vi "Immediate Shot Distance.vi"() -> (1 "Pointed At Goal?":bool, 2 "Aimpoint X":dbl, 3 "Aimpoint Distance":dbl)   [LabVIEW 2013]
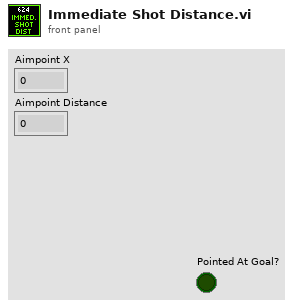
[diagram p1: front panel]
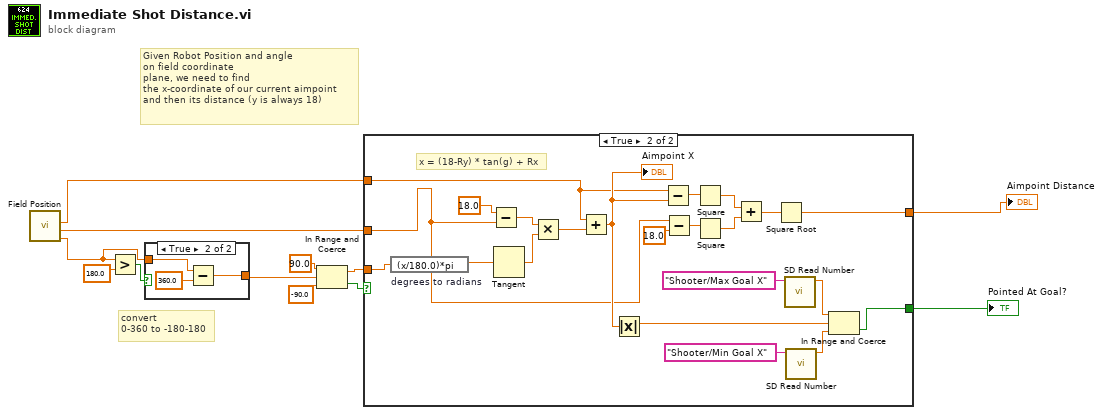
[diagram p0: block diagram]
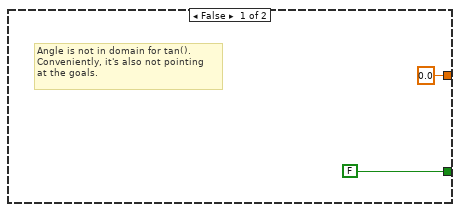
[diagram p2: hidden frame]
diagram:
  # "convert \n0-360 to -180-180"
  # "Given Robot Position and angle\non field coordinate\nplane, we need to find \nthe x-coordinate of our current aimpoint\nand then its distance (y is always 18)"
  n1 = call "Field Position.vi"() -> ("Field Angle"=w3:dbl, "Field Y"=w1:dbl, "Field X"=w2:dbl)  [unwired: 8 in, 1 out]
  n2 = Greater?(x=w3, y=180.0) -> (0:w11:bool)
  n3 = case shown="True" w11 {
    tunnel: w3 -> [w13 w16]
    tunnel: [w13 w14] -> w10
    frame False {
    }
    frame True {
      n4 = Subtract(x=w16, y=360.0) -> (x-y=w14:dbl)
    }
  }
  n5 = In Range and Coerce(upper limit=90.0, x=w10, lower limit=-90.0) -> (coerced(x)=w5:dbl, In Range?=w7:bool)
  n6 = case shown="True" w7 {
    tunnel: [FALSE w21] -> w6
    tunnel: w5 -> [_ w38]
    tunnel: [0.0 w27] -> w4
    tunnel: w2 -> [_ w20]
    tunnel: w1 -> [_ w19]
    frame False {
      # "Angle is not in domain for tan().\nConveniently, it's also not pointing\nat the goals."
    }
    frame True {
      # "x = (18-Ry) * tan(g) + Rx"
      n7 = expression code="(x/180.0)*pi" "degrees to radians"(w38) -> (w37:dbl)
      n8 = Subtract(x=18.0, y=w19) -> (x-y=w39:dbl)
      n9 = Tangent(1:w37) -> (0:w36:dbl)
      n10 = Multiply(x=w39, y=w36) -> (x*y=w35:dbl)
      n11 = Add(x=w20, y=w35) -> (x+y=w34:dbl)
      "Aimpoint X" <- w34
      n12 = Absolute Value(x=w34) -> (abs(x)=w24:dbl)
      n13 = Subtract(x=w20, y=w34) -> (x-y=w31:dbl)
      n14 = Subtract(x=w19, y=18.0) -> (x-y=w32:dbl)
      n15 = Square(x=w31) -> (x^2=w30:dbl)
      n16 = Square(x=w32) -> (x^2=w29:dbl)
      n17 = Add(x=w30, y=w29) -> (x+y=w28:dbl)
      n18 = Square Root(x=w28) -> (sqrt(x)=w27:dbl)
      n19 = call <vilib>:"SD Read Number.vi"("Name"="Shooter/Max Goal X") -> ("Numeric"=w23:dbl)  [unwired: 8 in, 2 out]
      n20 = call <vilib>:"SD Read Number.vi"("Name"="Shooter/Min Goal X") -> ("Numeric"=w22:dbl)  [unwired: 8 in, 2 out]
      n21 = In Range and Coerce(upper limit=w23, x=w24, lower limit=w22) -> (In Range?=w21:bool)  [unwired: 1 out]
    }
  }
  "Pointed At Goal?" <- w6
  "Aimpoint Distance" <- w4
